vi "FindingRealPartWhenImagIsZero.vi"(1 "Initial Guess Real":dbl=1.2999999523162842 step=0.001 format="%.3f", 2 "Extinction ExtinctionUncertainity Size parameter and Number ofS sizes 2":T1={"Extinction"=[], "Extinction Uncertainty"=[], "Size parameters"=[], "Number ofSizes"=0.0, "GeometricCrossSection"=[], "Wave Length"=0.0, "SMPS Sizes"=[], "Concentration"=[], "Double Charge Correction"=FALSE, "Extincation Factor"=1.0, "Diameter Factor"=1.0, "Diameter Offset"=0.0, "Extinction Factor Flag"=FALSE, "Diameter Factor Flag"=FALSE, "Diameter Offset Flag"=FALSE, "Sizes"=[], "ExtinctionOrAbsorptionOrScattering"=0} {"ExtinctionOrAbsorptionOrScattering" scale=0.0..2.0}) -> (0 "Real":dbl=1.2999999523162842 step=0.001 format="%.3f")   [LabVIEW 2011]
uses:
  BaesDataTypeDefinition.ctl
  <vilib>/gmath/NumericalOptimization/stopping criteria.ctl
  <vilib>/gmath/NumericalOptimization/Downhill Simplex.vi
  <vilib>/gmath/NI_Gmath.lvlib
panel:
  out "number of function evaluations":i32
  in  "cluster":T2={"Imaginary or Real Part"=0.0, "Chi Square at Minimum"=0.0, "Extinction ExtinctionUncertainity Size parameter and Number ofS sizes"={"Extinction"=[], "Extinction Uncertainty"=[], "Size parameters"=[], "Number ofSizes"=0.0, "GeometricCrossSection"=[], "Wave Length"=0.0, "SMPS Sizes"=[], "Concentration"=[], "Double Charge Correction"=FALSE, "Extincation Factor"=1.0, "Diameter Factor"=1.0, "Diameter Offset"=0.0, "Extinction Factor Flag"=FALSE, "Diameter Factor Flag"=FALSE, "Diameter Offset Flag"=FALSE, "Sizes"=[], "ExtinctionOrAbsorptionOrScattering"=0}} {"Extinction ExtinctionUncertainity Size parameter and Number ofS sizes"."ExtinctionOrAbsorptionOrScattering" scale=0.0..2.0}
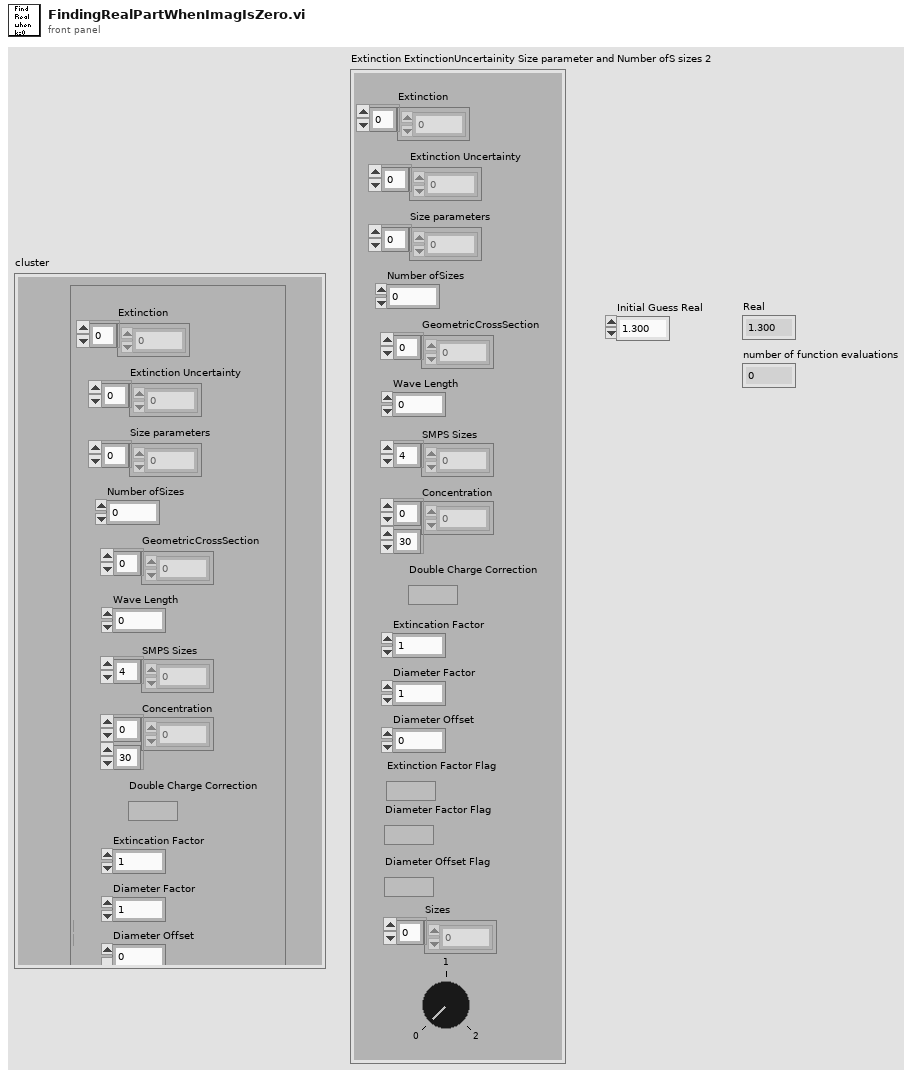
[diagram p1: front panel]
types:
  T1 = typedef "BaesDataTypeDefinition.ctl" = cluster{"Extinction":dbl[], "Extinction Uncertainty":dbl[], "Size parameters":dbl[], "Number ofSizes":dbl, "GeometricCrossSection":dbl[], "Wave Length":dbl, "SMPS Sizes":dbl[], "Concentration":dbl[][], "Double Charge Correction":bool, "Extincation Factor":dbl, "Diameter Factor":dbl, "Diameter Offset":dbl, "Extinction Factor Flag":bool, "Diameter Factor Flag":bool, "Diameter Offset Flag":bool, "Sizes":dbl[], "ExtinctionOrAbsorptionOrScattering":i8}
  T2 = cluster{"Imaginary or Real Part":dbl, "Chi Square at Minimum":dbl, "Extinction ExtinctionUncertainity Size parameter and Number ofS sizes":T1}
  T3 = typedef "NI_Gmath.lvlib/stopping criteria.ctl" = cluster{"function tolerance":dbl, "parameter tolerance":dbl, "max iterations":i32, "max function calls":i32, "gradient tolerance":dbl, "max time (sec)":dbl}
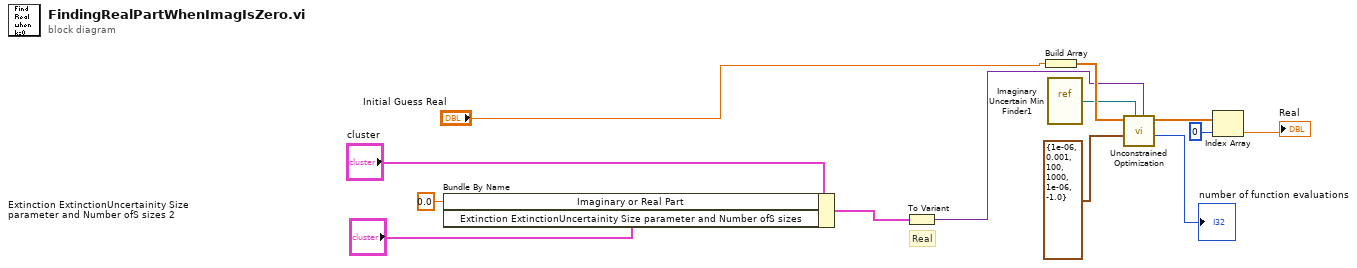
[diagram p0: block diagram]
diagram:
  # "Real"
  n1 = Bundle By Name(cluster="cluster", "Imaginary or Real Part"=0.0, "Extinction ExtinctionUncertainity Size parameter and Number ofS sizes"="Extinction ExtinctionUncertainity Size parameter and Number ofS sizes 2") -> (w13:T2)
  n2 = To Variant(anything=w13) -> (Variant=w10:variant)
  n3 = Build Array("Initial Guess Real") -> (w12:dbl[])
  n4 = vi-ref "Imaginary Uncertain Min Finder1.vi"() -> (w9:refnum<vi>)
  n5 = call-poly <vilib>:"Unconstrained Optimization.vi"("function data"=w10, "objective function"=w9, "stopping criteria"=T3 {"function tolerance"=1e-06, "parameter tolerance"=0.001, "max iterations"=100, "max function calls"=1000, "gradient tolerance"=1e-06, "max time (sec)"=-1.0}, "start"=w12) -> ("number of function evaluations"=→"number of function evaluations":i32, "minimum"=w8:dbl[])  [unwired: 4 in, 2 out]
  n6 = Index Array(array=w8, index=0) -> (element=→"Real":dbl)
